vi "Remove Duplicates.vi"(9 "Valid Pointer Names":string[](array[string]), 10 "Valid Pointer IDs":string[](array[string])) -> (1 "Valid Pointer Names out":string[](array[string]), 2 "Valid Pointer IDs out":string[](array[string]))   [LabVIEW 2017, in "Conditional Dialog.lvclass"]
uses:
  <vilib>/gpm_packages/@cs/Test-executive-builder/Source/Test Executive Builder Dialogs/Edit Conditional Dialog/Conditional Dialog.lvclass
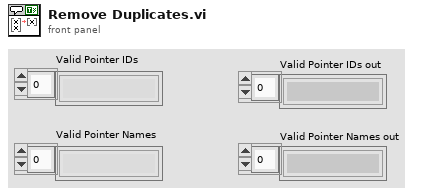
[diagram p1: front panel]
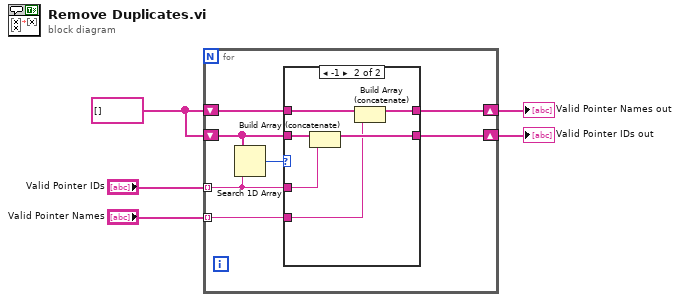
[diagram p0: block diagram]
diagram:
  w1 = string[] [] ("initialized array")
  n1 = for {
    tunnel: "Valid Pointer IDs" -> [w11] mode=indexing
    shift-right: [w10] -> w4
    shift-left: w1 -> [w9]
    shift-right: [w8] -> w3
    shift-left: w1 -> [w7]
    tunnel: "Valid Pointer Names" -> [w6] mode=indexing
    n2 = Search 1D Array(1D array=w9, element=w11) -> (index of element=w12:i32)  [unwired: 1 in]
    n3 = case shown="-1" w12 {
      tunnel: w11 -> [_ w20]
      tunnel: [w14 w18] -> w10
      tunnel: w9 -> [w14 w19]
      tunnel: [w13 w16] -> w8
      tunnel: w7 -> [w13 w17]
      tunnel: w6 -> [_ w15]
      frame Default {
      }
      frame -1 {
        n4 = Build Array (concatenate)(w19, w20) -> (w18:string[])
        n5 = Build Array (concatenate)(w17, w15) -> (w16:string[])
      }
    }
  }
  "Valid Pointer IDs out" <- w4
  "Valid Pointer Names out" <- w3
